vi "subHasBuildSpecifications.vi"(8 "error in (no error)":errorcluster, 11 "SolutionBuilder in":refnum<class "SolutionBuilder.lvclass">) -> (0 "error out":errorcluster, 2 "Has specs?":bool, 3 "SolutionBuilder out":refnum<class "SolutionBuilder.lvclass">)   [LabVIEW 2019, in "SolutionBuilder.lvlib" / "SolutionBuilder.lvclass"]
uses:
  SolutionBuilder.lvclass
  ProjectItem/ProjectItem.lvclass
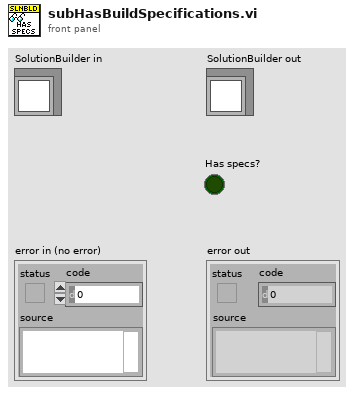
[diagram p1: front panel]
types:
  T1 = typedef "SolutionBuilder.lvlib/SolutionBuilder.lvclass/ProjectItemMap.ctl" = map{path, refnum<class "ProjectItem.lvclass">[]}
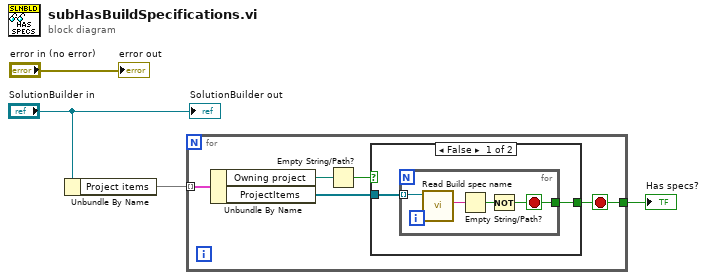
[diagram p0: block diagram]
diagram:
  n1 = Unbundle By Name("SolutionBuilder in") -> ("Project items"=w2:T1)
  n2 = for {
    tunnel: w2 -> [w9] mode=indexing
    tunnel: [w5] -> w1
    stop <- w5 stop-if-true
    n3 = Unbundle By Name(w9) -> ("Owning project"=w7:path, "ProjectItems"=w8:refnum<class "ProjectItem.lvclass">[])
    n4 = Empty String/Path?(string/path=w7) -> (empty?=w6:bool)
    n5 = case shown="False" w6 {
      tunnel: w8 -> [w11 _]
      tunnel: [w10 _] -> w5
      frame False {
        n6 = for {
          tunnel: w11 -> [w15] mode=indexing
          tunnel: [w12] -> w10
          stop <- w12 stop-if-true
          n7 = call-dynamic "Read Build spec name.vi"("ProjectItem in"=w15) -> ("Build spec name"=w14:string)  [unwired: 9 in, 1 out]
          n8 = Empty String/Path?(string/path=w14) -> (empty?=w13:bool)
          n9 = Not(x=w13) -> (.not. x?=w12:bool)
        }
      }
      frame True {
      }
    }
  }
  "Has specs?" <- w1
  "error out" <- "error in (no error)"
  "SolutionBuilder out" <- "SolutionBuilder in"
